vi "Get Enable Generic Event Flag.vi"(11 "Template Server in":refnum<class "Template Server.lvclass">) -> (2 "Enable Generic Event Flag":bool, 3 "Template Server out":refnum<class "Template Server.lvclass">)   [LabVIEW 2019, in "Template Server.lvlib" / "Template Server.lvclass"]
uses:
  Template Server.lvclass
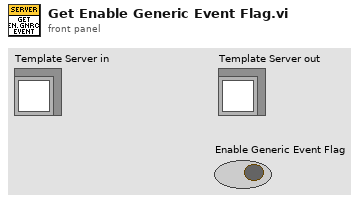
[diagram p1: front panel]
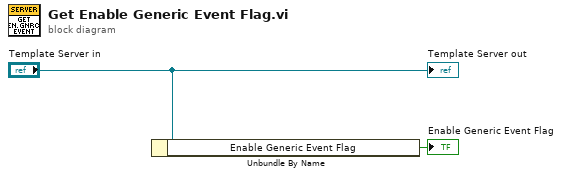
[diagram p0: block diagram]
diagram:
  n1 = Unbundle By Name("Template Server in") -> ("Enable Generic Event Flag"=→"Enable Generic Event Flag":bool)
  "Template Server out" <- "Template Server in"
